vi "Facade.vi"(0 "Data In":T7 {"octave info"."engineering units" items=["custom..."=0, "V"=1, "A"=21, "C"=30, "pC"=31, "s"=32, "-"=29, "Pa"=2, "N"=20, "g"=3, "m/s^2"=4, "m/s"=5, "m"=6, "mm/s"=12, "mm"=13, "micron/s"=14, "micron"=15, "in/s^2"=7, "in/s"=8, "in"=9, "mil/s"=10, "mil"=11, "rad/s^2"=16, "rad/s"=17, "rad"=18, "deg/s^2"=26, "deg/s"=27, "deg"=28, "RPM"=22, "cycle/s^2"=23, "Hz"=24, "cycle"=25, "strain"=19]; "octave info"."dB reference" format="%.2e"; "octave info"."weighting filter" items=["Linear", "A-weighting", "B-weighting", "C-weighting", "ITU-R 468-4", "Dolby", "CCITT", "C-message", "Wb", "Wc", "Wd", "We", "Wf", "Wh", "Wj", "Wk", "Wm", "AES17 20 kHz lowpass", "AES17 40 kHz lowpass", "AES17 20 kHz highpass", "AES17 40 kHz highpass"]; "octave spectra"."band power" format="%.2f"; "octave spectra"."nominal frequencies [Hz]" format="%.2f"}, 2 "Display State In":T3={"Graph Visible Items"={"Plot Legend"=FALSE, "Scale Legend"=FALSE, "Graph Palette"=FALSE, "Cursor Legend"=FALSE, "X Scrollbar"=FALSE}, "View Table"=FALSE, "Table Visible Items"={"Vertical Scrollbar"=FALSE, "Horizontal Scrollbar"=FALSE, "Row Headers"=FALSE, "Column Headers"=FALSE, "Vertical Lines"=FALSE, "Horizontal Lines"=FALSE}, "Header Font"={"Font Name"="", "Size"=0, "Bold"=FALSE, "Italic"=FALSE, "Underline"=FALSE, "Strikeout"=FALSE, "Color"=0}, "Cell Font"={"Font Name"="", "Size"=0, "Bold"=FALSE, "Italic"=FALSE, "Underline"=FALSE, "Strikeout"=FALSE, "Color"=0}, "Description and Tip..."={"Description"="", "Tip"=""}, "Moveable Splitter Position"=0, "Measurement Cursor Configuration"={"XY"={"enable XY"=FALSE, "Position (X)"=[], "Type"=enum."Absolute", "Y reference"=0.0, "color"=0}, "band"={"enable band"=FALSE, "B1"=0.0, "B2"=0.0, "Fixed bandwidth (B2-B1)"=0.0, "B1 color"=0, "B2 color"=0}, "harmonic"={"enable harmonics"=FALSE, "X reference (1X)"=0.0, "Maximum"=0, "Subset"=enum."All", "1X color"=0, "MX color"=0}, "sideband"={"enable sideband"=FALSE, "X center (C)"=0.0, "Sidebands"=0, "X spacing (s)"=0.0, "Center color"=0, "Sideband color"=0}}, "Cursors"={"List"=[], "Tags"=[]}, "X Increment"=0.0, "X Scale"={"Label Visible"=FALSE, "Label Text"="", "Mapping Mode"=0, "Format String"=""}, "Y Scale"={"Label Visible"=FALSE, "Label Text"="", "Mapping Mode"=0, "Format String"=""}, "Colors"={"background"=16777215, "major grid"=8355711, "minor grid"=12632256, "font"=0}, "desired spectrum view"={"scaling"={"linear/dB"=enum."no change", "dB reference"=0.0, "power/magnitude"=enum."no change", "view"=enum."no change"}, "spectral density"=enum."no change"}, "Plot Color Wheel"=[3381759, 32768, 982784, 4375295, 13827953, 13457919, 16757522, 4343295, 16728758, 12095254], "Plots"=[], "registered user events"=variant, "Lock 1X to Peak"=FALSE} {"Y Scale"."Mapping Mode" items=["Linear", "Logarithmic", "dB"]; "X Scale"."Mapping Mode" items=["Linear", "Logarithmic"]}, 3 "Container State":T6) -> (6 "Data Out":T7 {"octave info"."engineering units" items=["custom..."=0, "V"=1, "A"=21, "C"=30, "pC"=31, "s"=32, "-"=29, "Pa"=2, "N"=20, "g"=3, "m/s^2"=4, "m/s"=5, "m"=6, "mm/s"=12, "mm"=13, "micron/s"=14, "micron"=15, "in/s^2"=7, "in/s"=8, "in"=9, "mil/s"=10, "mil"=11, "rad/s^2"=16, "rad/s"=17, "rad"=18, "deg/s^2"=26, "deg/s"=27, "deg"=28, "RPM"=22, "cycle/s^2"=23, "Hz"=24, "cycle"=25, "strain"=19]; "octave info"."dB reference" format="%.2e"; "octave info"."weighting filter" items=["Linear", "A-weighting", "B-weighting", "C-weighting", "ITU-R 468-4", "Dolby", "CCITT", "C-message", "Wb", "Wc", "Wd", "We", "Wf", "Wh", "Wj", "Wk", "Wm", "AES17 20 kHz lowpass", "AES17 40 kHz lowpass", "AES17 20 kHz highpass", "AES17 40 kHz highpass"]; "octave spectra"."band power" format="%.2f"; "octave spectra"."nominal frequencies [Hz]" format="%.2f"}, 7 "Display State Out":T3={"Graph Visible Items"={"Plot Legend"=FALSE, "Scale Legend"=FALSE, "Graph Palette"=FALSE, "Cursor Legend"=FALSE, "X Scrollbar"=FALSE}, "View Table"=FALSE, "Table Visible Items"={"Vertical Scrollbar"=FALSE, "Horizontal Scrollbar"=FALSE, "Row Headers"=FALSE, "Column Headers"=FALSE, "Vertical Lines"=FALSE, "Horizontal Lines"=FALSE}, "Header Font"={"Font Name"="", "Size"=0, "Bold"=FALSE, "Italic"=FALSE, "Underline"=FALSE, "Strikeout"=FALSE, "Color"=0}, "Cell Font"={"Font Name"="", "Size"=0, "Bold"=FALSE, "Italic"=FALSE, "Underline"=FALSE, "Strikeout"=FALSE, "Color"=0}, "Description and Tip..."={"Description"="", "Tip"=""}, "Moveable Splitter Position"=0, "Measurement Cursor Configuration"={"XY"={"enable XY"=FALSE, "Position (X)"=[], "Type"=enum."Absolute", "Y reference"=0.0, "color"=0}, "band"={"enable band"=FALSE, "B1"=0.0, "B2"=0.0, "Fixed bandwidth (B2-B1)"=0.0, "B1 color"=0, "B2 color"=0}, "harmonic"={"enable harmonics"=FALSE, "X reference (1X)"=0.0, "Maximum"=0, "Subset"=enum."All", "1X color"=0, "MX color"=0}, "sideband"={"enable sideband"=FALSE, "X center (C)"=0.0, "Sidebands"=0, "X spacing (s)"=0.0, "Center color"=0, "Sideband color"=0}}, "Cursors"={"List"=[], "Tags"=[]}, "X Increment"=0.0, "X Scale"={"Label Visible"=FALSE, "Label Text"="", "Mapping Mode"=0, "Format String"=""}, "Y Scale"={"Label Visible"=FALSE, "Label Text"="", "Mapping Mode"=0, "Format String"=""}, "Colors"={"background"=16777215, "major grid"=8355711, "minor grid"=12632256, "font"=0}, "desired spectrum view"={"scaling"={"linear/dB"=enum."no change", "dB reference"=0.0, "power/magnitude"=enum."no change", "view"=enum."no change"}, "spectral density"=enum."no change"}, "Plot Color Wheel"=[3381759, 32768, 982784, 4375295, 13827953, 13457919, 16757522, 4343295, 16728758, 12095254], "Plots"=[], "registered user events"=variant, "Lock 1X to Peak"=FALSE} {"Y Scale"."Mapping Mode" items=["Linear", "Logarithmic", "dB"]; "X Scale"."Mapping Mode" items=["Linear", "Logarithmic"]}, 8 "Action":T2)   [LabVIEW 2017, in "Octave with Cursors.xctl"]
doc: "This is the facade VI for the Spectral Graph with Measurement Cursors XControl.\nThe facade VI is only used within the context of the XControl."
uses:
  <vilib>/addons/_XControls/Octave with Cursors/Octave with Cursors.xctl
  <vilib>/addons/_XControls/Octave with Cursors/Controls/Data.ctl
  <vilib>/addons/_NISVFA/_Shared subVIs/Controls/svc_Octave Info.ctl
  <vilib>/addons/_NISVFA/_Shared subVIs/Controls/svc_Octave Standard.ctl
  <vilib>/addons/_NISVFA/_Shared subVIs/Controls/svc_Weighting Filter Text Ring.ctl
  <vilib>/addons/_NISVFA/_Shared subVIs/Controls/svc_Engineering Units Text Ring.ctl
  <vilib>/_xctls/Container State.ctl
  <vilib>/addons/_XControls/Octave with Cursors/Controls/State.ctl
  <vilib>/Utility/miscctls.llb/LVFontTypeDef.ctl
  <vilib>/addons/_XControls/Octave with Cursors/Controls/Measurement Cursor Configuration.ctl
  <vilib>/_xctls/Action.ctl
  <vilib>/addons/Sound and Vibration/svt_Controls/subVIs/Multiplot Octave Graph.ctl
  <vilib>/addons/_XControls/Octave with Cursors/Controls/Refnums Typedef.ctl
  <vilib>/addons/_XControls/Octave with Cursors/Controls/Spectrum XControl Events.ctl
  <vilib>/Utility/miscctls.llb/LVForegroundBackgroundColorsTypeDef.ctl
  <vilib>/addons/Sound and Vibration/svt_Octave/SVT Octave Spectrum Conversion (N Ch).vi
  <vilib>/_xctls/XControlSupport.lvlib
  <vilib>/addons/Sound and Vibration/svt_Octave/SoundVib_Octave.lvlib
panel:
  out "plot names":string[](array[string])
  in  "Focus Boolean":bool
  out "Octave graph":T1
  in  "View Table":bool=TRUE
  in  "Cursor Table":string[][](table)
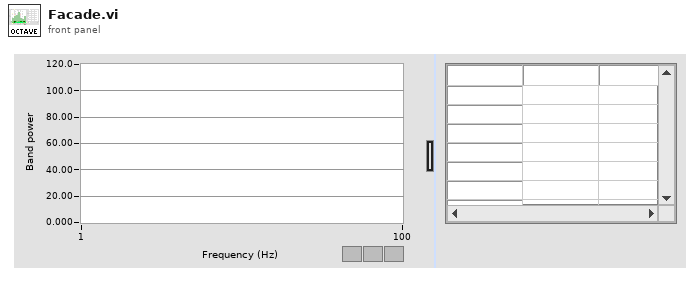
[diagram p1: front panel]
types:
  T1 = typedef "Multiplot Octave Graph.ctl" = cluster{"nominal frequencies [Hz]":dbl[], "band power [dB EU]":dbl[]}[]
  T2 = typedef "XControlSupport.lvlib/Action.ctl" = cluster{"Data Changed?":bool, "State Changed?":bool, "Action Name":string}
  T3 = typedef "Octave with Cursors.xctl/State.ctl" = cluster{"Graph Visible Items":cluster{"Plot Legend":bool, "Scale Legend":bool, "Graph Palette":bool, "Cursor Legend":bool, "X Scrollbar":bool}, "View Table":bool, "Table Visible Items":cluster{"Vertical Scrollbar":bool, "Horizontal Scrollbar":bool, "Row Headers":bool, "Column Headers":bool, "Vertical Lines":bool, "Horizontal Lines":bool}, "Header Font":T4, "Cell Font":T4, "Description and Tip...":cluster{"Description":string, "Tip":string}, "Moveable Splitter Position":i32, "Measurement Cursor Configuration":T5, "Cursors":cluster{"List":cluster{"Name":string, "Color":u32, "Style":i32, "Point Style":u8, "Name Visible":bool, "Allow Drag":bool, "Cursor Mode":u32, "Plot":i32, "Index":i32, "Position":cluster{"X":dbl, "Y":dbl}, "X Scale":u32, "Y Scale":u32, "Watch Plots":i32[], "Watch All Plots":bool, "Plot Area":i32, "Label Offset":cluster{"X":dbl, "Y":dbl}}[], "Tags":variant[]}, "X Increment":dbl, "X Scale":cluster{"Label Visible":bool, "Label Text":string, "Mapping Mode":u8, "Format String":string}, "Y Scale":cluster{"Label Visible":bool, "Label Text":string, "Mapping Mode":u8, "Format String":string}, "Colors":cluster{"background":u32, "major grid":u32, "minor grid":u32, "font":u32}, "desired spectrum view":cluster{"scaling":cluster{"linear/dB":enum16{"no change", "linear", "dB"}, "dB reference":dbl, "power/magnitude":enum16{"no change", "power", "magnitude"}, "view":enum16{"no change", "rms", "peak", "peak-peak"}}, "spectral density":enum16{"no change", "spectrum", "spectral density"}}, "Plot Color Wheel":u32[], "Plots":cluster{"Name":string, "Line Color":u32, "Line Style":u8, "Line Width":u8, "Fill/Point Color":u32, "Point Style":u8, "Fill To":i16, "Interpolation":u8, "Anti-aliased":bool}[], "registered user events":variant, "Lock 1X to Peak":bool}
  T4 = typedef "LVFontTypeDef.ctl" = cluster{"Font Name":string, "Size":u16, "Bold":bool, "Italic":bool, "Underline":bool, "Strikeout":bool, "Color":u32}
  T5 = typedef "Octave with Cursors.xctl/Measurement Cursor Configuration.ctl" = cluster{"XY":cluster{"enable XY":bool, "Position (X)":dbl[], "Type":enum16{"Absolute", "Relative"}, "Y reference":dbl, "color":u32}, "band":cluster{"enable band":bool, "B1":dbl, "B2":dbl, "Fixed bandwidth (B2-B1)":dbl, "B1 color":u32, "B2 color":u32}, "harmonic":cluster{"enable harmonics":bool, "X reference (1X)":dbl, "Maximum":i32, "Subset":enum16{"All", "Even", "Odd"}, "1X color":u32, "MX color":u32}, "sideband":cluster{"enable sideband":bool, "X center (C)":dbl, "Sidebands":i32, "X spacing (s)":dbl, "Center color":u32, "Sideband color":u32}}
  T6 = typedef "XControlSupport.lvlib/Container State.ctl" = cluster{"Indicator?":bool, "Run Mode?":bool, " Refnum":refnum<vi>}
  T7 = typedef "Octave with Cursors.xctl/Data.ctl" = cluster{"octave spectra":cluster{"nominal frequencies [Hz]":dbl[], "band power":dbl[]}[], "octave info":T8[]}
  T8 = typedef "svc_Octave Info.ctl" = cluster{"standard":T9, "bandwidth":enum16{"1 octave", "1/3 octave", "1/6 octave", "1/12 octave", "1/24 octave"}, "low band":i32, "high band":i32, "weighting filter":T10, "dB reference":dbl, "dB On":bool, "unit label":string, "channel name":string, "description":string, "engineering units":T11, "custom label":string, "spectrum type":enum16{"power", "magnitude"}, "spectral density":bool, "filters settled":bool}
  T9 = typedef "svc_Octave Standard.ctl" = enum16{"ANSI S1.11", "IEC 61260"}
  T10 = typedef "svc_Weighting Filter Text Ring.ctl" = u16
  T11 = typedef "svc_Engineering Units Text Ring.ctl" = u16
  T12 = typedef "Octave with Cursors.xctl/Refnums Typedef.ctl" = cluster{"Facade Panel Refnum":refnum<vi>, "Splitters":cluster{"Moveable":refnum<vi>, "Locked":refnum<vi>}, "Panes":cluster{"Container":refnum<vi>, "Graph":refnum<vi>, "Table":refnum<vi>, "Fixed-Width":refnum<vi>}, "Controls":cluster{"XYGraph":refnum<vi>, "Table":refnum<vi>, "View Table":refnum<vi>, "Focus Boolean":refnum<vi>, "Plot Names":refnum<vi>}}
  T13 = typedef "Octave with Cursors.xctl/Spectrum XControl Events.ctl" = string
  T14 = cluster{"linear/dB":enum16{"no change", "linear", "dB"}, "dB reference (0: no change)":dbl, "power/magnitude":enum16{"no change", "power", "magnitude"}, "spectral density":enum16{"no change", "spectrum", "spectral density"}}
  T15 = typedef "LVForegroundBackgroundColorsTypeDef.ctl" = cluster{"Foreground Color":u32, "Background Color":u32}
  T16 = cluster{"nominal frequencies [Hz]":dbl[], "band power":dbl[]}[]
  T17 = cluster{"nominal frequencies [Hz]":dbl[], "band power":dbl[]}
  T18 = typedef "eventvkey.ctl" = enum16{"ASCII", "Enter", "Return", "Shift", "Ctrl", "Alt", "Cmd", "Opt", "Caps", "NumLock", "Clear", "Break", "Up", "Down", "Left", "Right", "Insert", "Delete", "Home", "End", "PageUp", "PageDown", "Escape", "Help", "Pause", "ScrollLock", "F1", "F2", "F3", "F4", "F5", "F6", "F7", "F8", "F9", "F10", "F11", "F12", "F13", "F14", "F15", "F16", "F17", "F18", "F19", "F20", "F21", "F22", "F23", "F24", "Play", "VolumeUp", "VolumeDown", "Mute", "Two Byte Char"}
  T19 = cluster{"Shift":bool, "Ctrl":bool, "Alt":bool, "Cmd":bool, "Opt":bool}
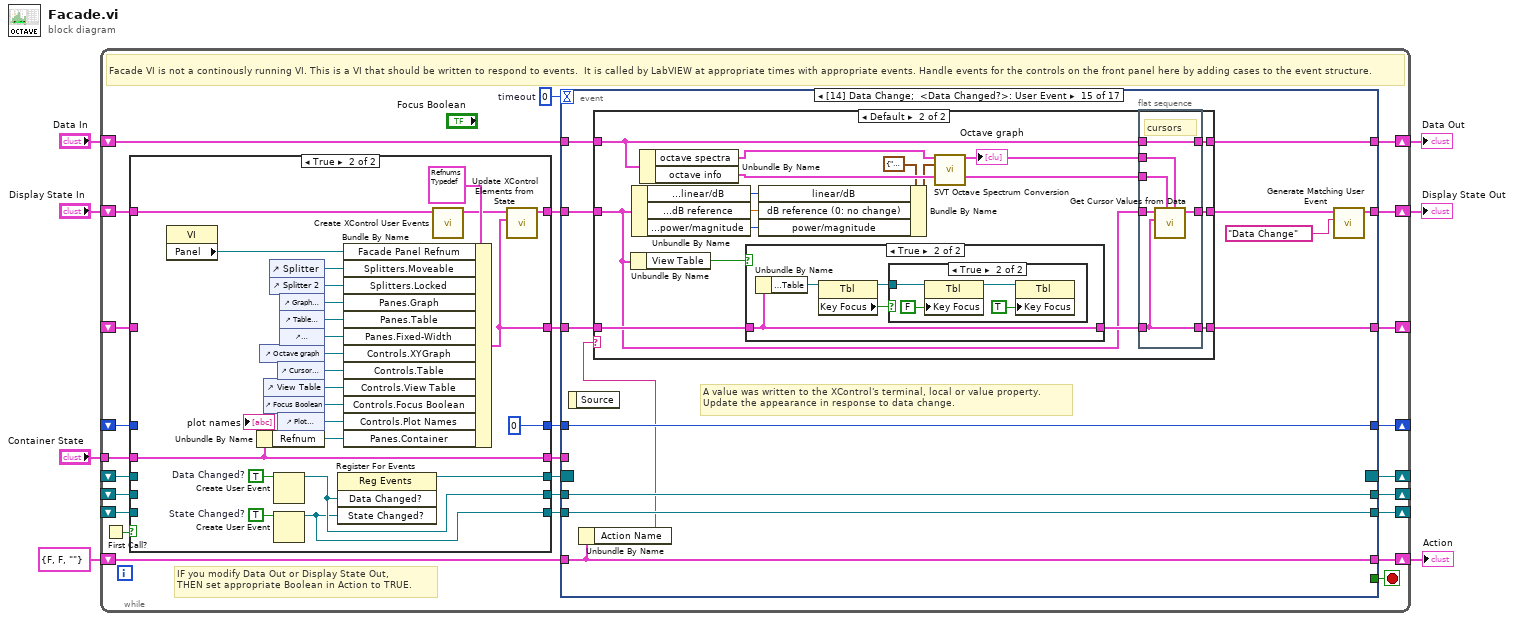
[diagram p0: block diagram]
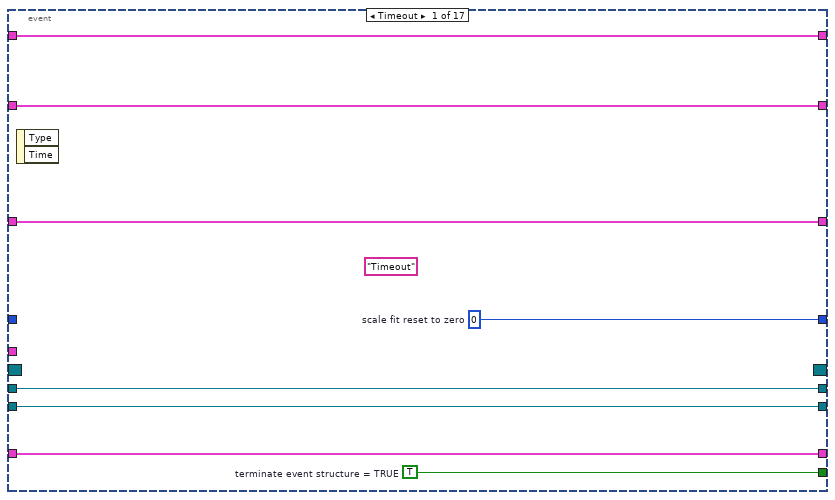
[diagram p3: hidden frame]
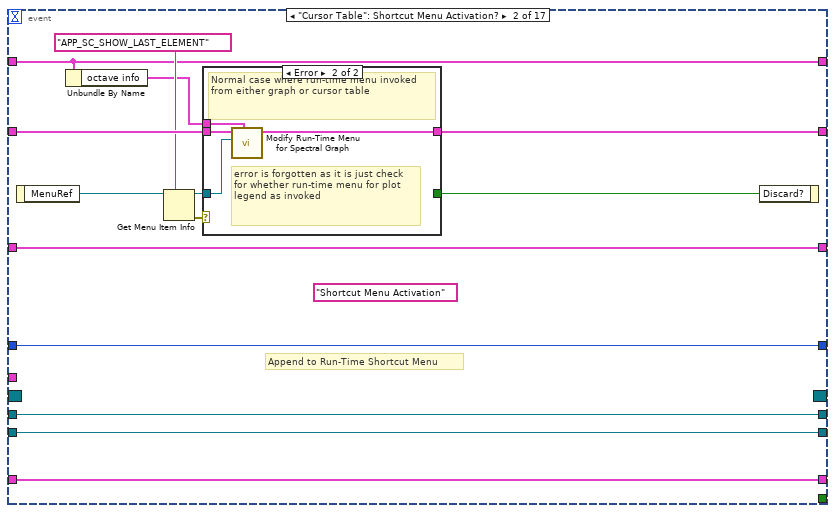
[diagram p4: hidden frame]
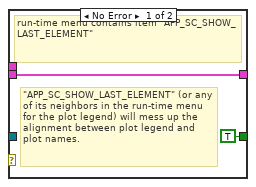
[diagram p5: hidden frame]
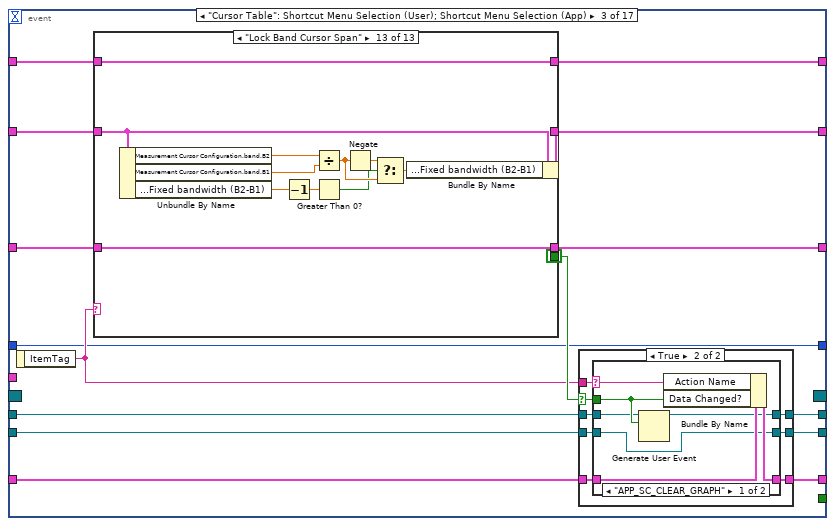
[diagram p6: hidden frame]
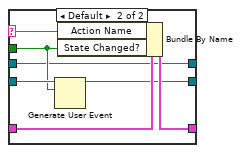
[diagram p8: hidden frame]
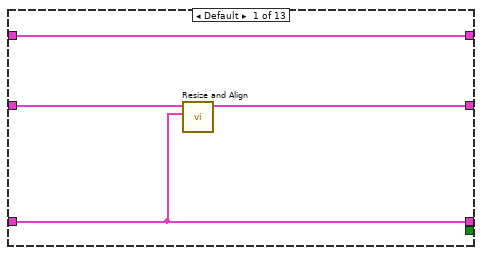
[diagram p9: hidden frame]
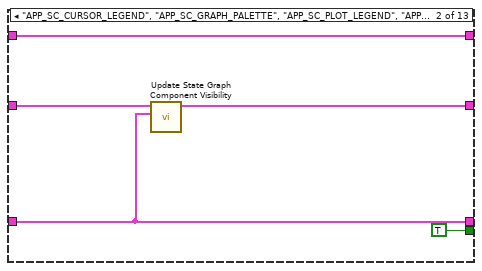
[diagram p10: hidden frame]
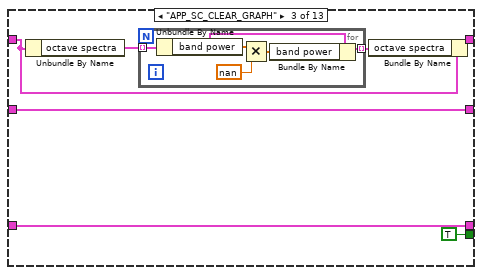
[diagram p11: hidden frame]
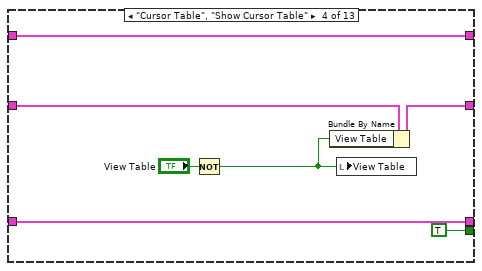
[diagram p12: hidden frame]
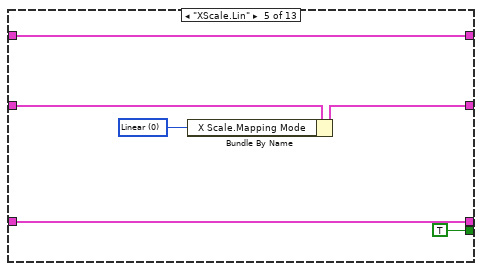
[diagram p13: hidden frame]
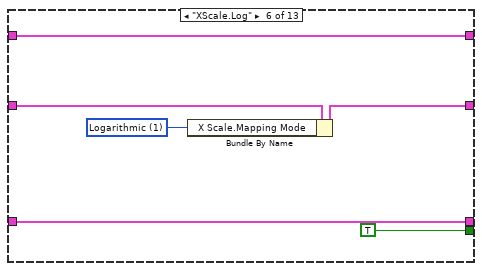
[diagram p14: hidden frame]
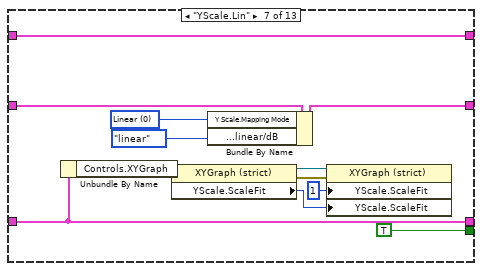
[diagram p15: hidden frame]
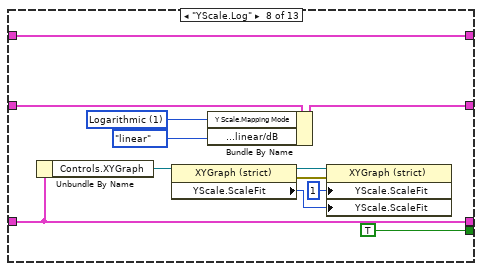
[diagram p16: hidden frame]
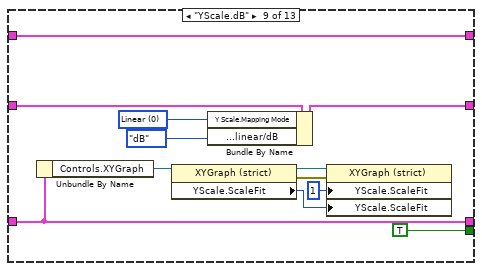
[diagram p17: hidden frame]
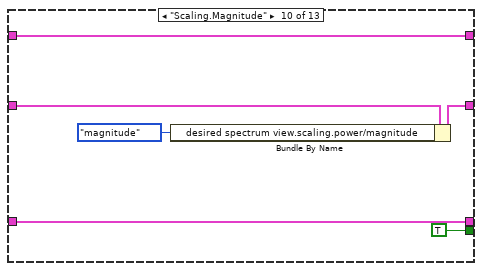
[diagram p18: hidden frame]
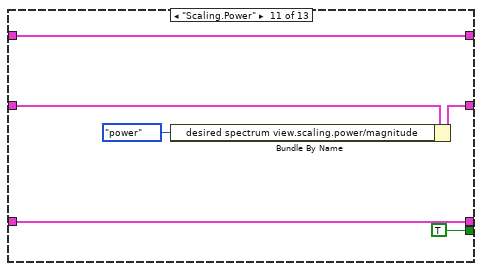
[diagram p19: hidden frame]
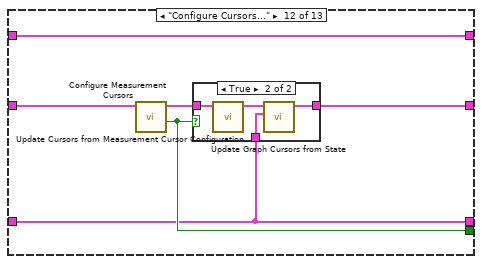
[diagram p20: hidden frame]
diagram:
  n1 = while {
    shift-right: [w28] -> w5
    shift-left: "Display State In" -> [w12]
    tunnel: "Container State" -> [w18]
    shift-right: [w32] -> w7
    shift-left: "Data In" -> [w29]
    shift-right: [w30] -> w2
    shift-left: T2 {"Data Changed?"=FALSE, "State Changed?"=FALSE, "Action Name"=""} ("Action") -> [w31]
    shift-right: [w25] -> _
    shift-left: _ -> [w23]
    shift-right: [w20] -> _
    shift-left: _ -> [w19]
    shift-right: [w24] -> _
    shift-left: _ -> [w21]
    shift-right: [w13] -> _
    shift-left: _ -> [w15]
    shift-right: [w10] -> _
    shift-left: _ -> [w9]
    stop <- w34 stop-if-true
    w33 = 0  # timeout
    # "IF you modify Data Out or Display State Out, \nTHEN set appropriate Boolean in Action to TRUE."
    # "Facade VI is not a continously running VI. This is a VI that should be written to respond to events.  It is called by LabVIEW at appropriate times with appropriate events. Handle events for the controls on the front panel here by adding cases to the event structure."
    n2 = First Call?() -> (First Call?: T/F=w22:bool)
    n3 = case shown="True" w22 {
      tunnel: [w41 w54] -> w14
      tunnel: [w40 w55] -> w27
      tunnel: [w39 w56] -> w26
      tunnel: w23 -> [w41 _]
      tunnel: w21 -> [w40 _]
      tunnel: w19 -> [w39 _]
      tunnel: w18 -> [w37 w50]
      tunnel: [w37 w50] -> w17
      tunnel: [w38 w46] -> w16
      tunnel: w15 -> [w38 _]
      tunnel: w12 -> [w35 w49]
      tunnel: [w35 w47] -> w11
      tunnel: [w36 u8 0 ("Scale Fit")] -> w8
      tunnel: w9 -> [w36 _]
      frame False {
      }
      frame True {
        w65 = TRUE  # State Changed?
        w64 = TRUE  # Data Changed?
        n4 = property class="VI"() -> ("Panel"=w45:refnum<vi>)  [unwired: 2 in, 2 out]
        n5 = Unbundle By Name(w50) -> ("Refnum"=w52:refnum<vi>)
        n6 = control-ref of="Octave graph"() -> (w43:refnum<vi>)
        n7 = control-ref of="View Table"() -> (w59:refnum<vi>)
        n8 = control-ref of="Focus Boolean"() -> (w53:refnum<vi>)
        n9 = control-ref of="Splitter"() -> (w58:refnum<vi>)
        n10 = control-ref of="Splitter 2"() -> (w57:refnum<vi>)
        n11 = Create User Event(user event datatype=w64) -> (user event=w56:refnum<user-event>)  [unwired: 1 in, 1 out]
        n12 = Create User Event(user event datatype=w65) -> (user event=w55:refnum<user-event>)  [unwired: 1 in, 1 out]
        n13 = control-ref of="Cursor Table"() -> (w60:refnum<vi>)
        n14 = control-ref of="Plot Names"() -> (w51:refnum<vi>)
        n15 = control-ref of="Graph Pane"() -> (w42:refnum<vi>)
        n16 = control-ref of="Table Pane"() -> (w62:refnum<vi>)
        n17 = control-ref of="Fixed-Width Pane"() -> (w61:refnum<vi>)
        n18 = register-events(w56, w55) -> (reference out=w54:refnum<event-registration>)  [unwired: 2 in, 1 out]
        n19 = Bundle By Name(cluster=T12 {"Facade Panel Refnum"=refnum, "Splitters"={"Moveable"=refnum, "Locked"=refnum}, "Panes"={"Container"=refnum, "Graph"=refnum, "Table"=refnum, "Fixed-Width"=refnum}, "Controls"={"XYGraph"=refnum, "Table"=refnum, "View Table"=refnum, "Focus Boolean"=refnum, "Plot Names"=refnum}} ("Refnums for Resizing and Alignment"), "Facade Panel Refnum"=w45, "Splitters.Moveable"=w58, "Splitters.Locked"=w57, "Panes.Graph"=w42, "Panes.Table"=w62, "Panes.Fixed-Width"=w61, "Controls.XYGraph"=w43, "Controls.Table"=w60, "Controls.View Table"=w59, "Controls.Focus Boolean"=w53, "Controls.Plot Names"=w51, "Panes.Container"=w52) -> (w46:T12)
        n20 = call <vilib>:"Create XControl User Events.vi"("Display State In in"=w49) -> ("Display State In out"=w44:T3)  [unwired: 9 in, 1 out]
        n21 = call <vilib>:"Update XControl Elements from State.vi"("Refnums for FP Objects"=w46, "State in"=w44) -> ("State out"=w47:T3)  [unwired: 9 in]
      }
    }
    n22 = event shown="[14] Data Change;  <Data Changed?>: User Event" {
      selector: w14 -> [_ _ _ _ _ _ _ _ _ _ _ _ _ _ _ _ _]
      dyn-events: [_ _ _ _ _ _ _ _ _ _ _ _ _ _ _ _ _] -> w25
      timeout: w33 -> [_ _ _ _ _ _ _ _ _ _ _ _ _ _ _ _ _]
      tunnel: w11 -> [w71 w83 w108 w249 w275 w286 w317 w349 w364 w377 w419 w457 w492 w508 w542 w601 w609]
      tunnel: [w71 w82 w107 w246 w274 w285 w316 w333 w363 w380 w421 w459 w491 w509 w547 w601 w609] -> w28
      tunnel: [w73 _ _ _ _ _ _ _ _ _ _ _ _ _ _ _ _] -> w34
      tunnel: w17 -> [_ _ _ _ _ _ _ _ _ _ _ _ _ _ _ w602 w610]
      tunnel: w29 -> [w70 w75 w94 w267 w284 w295 w321 w350 w368 w389 w429 w467 w497 w513 w553 w600 w608]
      tunnel: [w70 w75 w95 w267 w284 w295 w321 w350 w368 w389 w429 w467 w497 w513 w552 w600 w608] -> w32
      tunnel: [w72 w87 w105 w263 w279 w294 w320 w347 w367 w387 w427 w465 w496 w502 w544 w599 w607] -> w30
      tunnel: w31 -> [w72 w87 w106 w264 w280 w294 w320 w348 w367 w388 w428 w466 w496 w503 w544 w599 w607]
      tunnel: w16 -> [w67 w84 w100 w250 w283 w288 w318 w337 w362 w375 w417 w456 w493 w507 w546 w592 w604]
      tunnel: w26 -> [w69 w86 w101 w262 w278 w292 w313 w342 w365 w383 w423 w461 w494 w512 w545 w596 w606]
      tunnel: w27 -> [w68 w85 w104 w261 w277 w293 w312 w345 w366 w386 w426 w464 w495 w500 w543 w595 w605]
      tunnel: [w68 w85 w103 w260 w276 w293 w312 w344 w366 w385 w425 w463 w495 w499 w543 w595 w605] -> w24
      tunnel: [w69 w86 w102 w262 w278 w292 w313 w343 w365 w384 w424 w462 w494 w511 w545 w596 w606] -> w20
      tunnel: [w67 w84 w99 w250 w283 w287 w318 w337 w362 w375 w417 w456 w493 w505 w549 w592 w604] -> w13
      tunnel: [w66 w81 w96 w247 w272 w289 w310 w334 w361 w369 w410 w448 w486 w504 w551 w591 w603] -> w10
      tunnel: w8 -> [_ w81 w96 w247 w272 _ w311 w334 w361 w369 w410 w448 w486 w504 w551 w591 w603]
      event Timeout {
        w66 = u8 0  # scale fit reset to zero
        (unwired) "Timeout"
        w73 = TRUE  # terminate event structure = TRUE
        n23 = event-data() -> ()  [unwired: 1 in, 2 out]
      }
      event "Cursor Table": Shortcut Menu Activation? {
        (unwired) "Shortcut Menu Activation"
        # "Append to Run-Time Shortcut Menu"
        n24 = event-data() -> ("MenuRef"=w80:refnum<k9>)  [unwired: 1 in]
        n25 = Unbundle By Name(w75) -> ("octave info"=w74:T8[])
        n26 = Get Menu Item Info(7:"APP_SC_SHOW_LAST_ELEMENT", 11:w80) -> (0:w77:errorcluster, 3:w79:refnum<k9>)  [unwired: 1 in, 5 out]
        n27 = case shown="Error" w77 {
          tunnel: w83 -> [w89 w93]
          tunnel: [w89 w92] -> w82
          tunnel: w79 -> [_ w91]
          tunnel: [TRUE _] -> w76
          tunnel: w74 -> [_ w90]
          frame No Error {
            # "\"APP_SC_SHOW_LAST_ELEMENT\" (or any of its neighbors in the run-time menu for the plot legend) will mess up the alignment between plot legend and plot names."
            # "run-time menu contains item \"APP_SC_SHOW_LAST_ELEMENT\""
          }
          frame Error {
            # "error is forgotten as it is just check for whether run-time menu for plot legend as invoked"
            # "Normal case where run-time menu invoked from either graph or cursor table"
            n28 = call <vilib>:"Modify Run-Time Menu for Spectral Graph.vi"("octave info"=w90, "Menu in"=w91, "Display State In"=w93) -> ("Display State out"=w92:T3)  [unwired: 8 in]
          }
        }
        n29 = event-data("Discard?"=w76) -> ()  [unwired: 1 in, 1 out]
      }
      event "Cursor Table": Shortcut Menu Selection (User); Shortcut Menu Selection (App) {
        n30 = event-data() -> ("ItemTag"=w97:string)  [unwired: 1 in]
        n31 = case shown="\"Lock Band Cursor Span\"" w97 {
          tunnel: w108 -> [w137 w142 w149 w159 w166 w173 w185 w197 w209 w214 w220 w227 w237]
          tunnel: [w136 w141 w149 w158 w165 w172 w184 w196 w208 w213 w219 w225 w236] -> w107
          tunnel: [_ TRUE ("state changed") TRUE ("state changed") TRUE ("state changed") TRUE ("state changed") TRUE ("state changed") TRUE ("state changed") TRUE ("state changed") TRUE ("state changed") TRUE ("state changed") TRUE ("state changed") w224 TRUE ("state changed")] -> w98
          tunnel: w100 -> [w135 w140 w148 w161 w167 w169 w175 w187 w199 w215 w221 w223 w245]
          tunnel: [w135 w140 w148 w161 w167 w169 w175 w187 w199 w215 w221 w223 w245] -> w99
          tunnel: [w134 w138 w144 w155 w162 w168 w174 w186 w198 w210 w216 w222 w234] -> w95
          tunnel: w94 -> [w134 w138 w143 w155 w162 w168 w174 w186 w198 w210 w216 w222 w234]
          frame Default {
            n32 = call <vilib>:"Resize and Align.vi"("Refnums for Resizing and Alignment"=w135, "State in"=w137) -> ("State out"=w136:T3)  [unwired: 8 in, 1 out]
          }
          frame "APP_SC_CURSOR_LEGEND", "APP_SC_GRAPH_PALETTE", "APP_SC_PLOT_LEGEND", "APP_SC_SCALE_LEGEND", "APP_SC_X_SCALE", "APP_SC_X_SCROLLBAR", "APP_SC_Y_SCALE" {
            n33 = call <vilib>:"Update State Graph Component Visibility.vi"("Refnums for FP Objects"=w140, "State in"=w142) -> ("State out"=w141:T3)  [unwired: 9 in]
          }
          frame "APP_SC_CLEAR_GRAPH" {
            n34 = Unbundle By Name(w143) -> ("octave spectra"=w146:T16)
            n35 = for {
              tunnel: w146 -> [w152] mode=indexing
              tunnel: [w150] -> w145 mode=indexing
              n36 = Unbundle By Name(w152) -> ("band power"=w154:dbl[])
              n37 = Multiply(x=w154, y=nan) -> (x*y=w151:dbl[])
              n38 = Bundle By Name(cluster=w152, "band power"=w151) -> (w150:T17)
            }
            n39 = Bundle By Name(cluster=w143, "octave spectra"=w145) -> (w144:T7)
          }
          frame "Cursor Table", "Show Cursor Table" {
            n40 = Not(x="View Table") -> (.not. x?=w157:bool)
            n41 = Bundle By Name(cluster=w159, "View Table"=w157) -> (w158:T3)
            n42 = local write "View Table"(w157) -> ()
          }
          frame "XScale.Lin" {
            w163 = u8 0 items=["Linear", "Logarithmic"] ("Mapping Mode")
            n43 = Bundle By Name(cluster=w166, "X Scale.Mapping Mode"=w163) -> (w165:T3)
          }
          frame "XScale.Log" {
            w171 = u8 1 items=["Linear", "Logarithmic"] ("Mapping Mode")
            n44 = Bundle By Name(cluster=w173, "X Scale.Mapping Mode"=w171) -> (w172:T3)
          }
          frame "YScale.Lin" {
            w183 = u8 0 items=["Linear", "Logarithmic"] ("Mapping Mode")
            n45 = Unbundle By Name(w175) -> ("Controls.XYGraph"=w176:refnum<vi>)
            n46 = property class="XYGraph (strict)"(reference=w176) -> (reference out=w177:refnum<vi>, error out=w178:errorcluster, "YScale.ScaleFit"=w179:u8)  [unwired: 1 in]
            n47 = Bundle By Name(cluster=w185, "Y Scale.Mapping Mode"=w183, "desired spectrum view.scaling.linear/dB"=enum16{"no change", "linear", "dB"}."linear" ("spectrum view.desired scaling.linear/dB")) -> (w184:T3)
            n48 = property class="XYGraph (strict)"(reference=w177, error in=w178, "YScale.ScaleFit"=u8 1 ("Y Scale.Scale Fit"), "YScale.ScaleFit"=w179) -> ()  [unwired: 2 out]
          }
          frame "YScale.Log" {
            w194 = u8 1 items=["Linear", "Logarithmic"] ("Mapping Mode")
            n49 = Unbundle By Name(w187) -> ("Controls.XYGraph"=w188:refnum<vi>)
            n50 = property class="XYGraph (strict)"(reference=w188) -> (reference out=w189:refnum<vi>, error out=w190:errorcluster, "YScale.ScaleFit"=w191:u8)  [unwired: 1 in]
            n51 = Bundle By Name(cluster=w197, "Y Scale.Mapping Mode"=w194, "desired spectrum view.scaling.linear/dB"=enum16{"no change", "linear", "dB"}."linear" ("spectrum view.desired scaling.linear/dB")) -> (w196:T3)
            n52 = property class="XYGraph (strict)"(reference=w189, error in=w190, "YScale.ScaleFit"=u8 1 ("Y Scale.Scale Fit"), "YScale.ScaleFit"=w191) -> ()  [unwired: 2 out]
          }
          frame "YScale.dB" {
            w206 = u8 0 items=["Linear", "Logarithmic"] ("Mapping Mode")
            n53 = Unbundle By Name(w199) -> ("Controls.XYGraph"=w200:refnum<vi>)
            n54 = property class="XYGraph (strict)"(reference=w200) -> (reference out=w201:refnum<vi>, error out=w202:errorcluster, "YScale.ScaleFit"=w203:u8)  [unwired: 1 in]
            n55 = Bundle By Name(cluster=w209, "Y Scale.Mapping Mode"=w206, "desired spectrum view.scaling.linear/dB"=enum16{"no change", "linear", "dB"}."dB" ("spectrum view.desired scaling.linear/dB")) -> (w208:T3)
            n56 = property class="XYGraph (strict)"(reference=w201, error in=w202, "YScale.ScaleFit"=u8 1 ("Y Scale.Scale Fit"), "YScale.ScaleFit"=w203) -> ()  [unwired: 2 out]
          }
          frame "Scaling.Magnitude" {
            n57 = Bundle By Name(cluster=w214, "desired spectrum view.scaling.power/magnitude"=enum16{"no change", "power", "magnitude"}."magnitude") -> (w213:T3)
          }
          frame "Scaling.Power" {
            n58 = Bundle By Name(cluster=w220, "desired spectrum view.scaling.power/magnitude"=enum16{"no change", "power", "magnitude"}."power") -> (w219:T3)
          }
          frame "Configure Cursors..." {
            n59 = call <vilib>:"Configure Measurement Cursors.vi"("State in"=w227) -> ("OK"=w224:bool, "State out"=w226:T3)  [unwired: 9 in]
            n60 = case shown="True" w224 {
              tunnel: w226 -> [w228 w232]
              tunnel: [w228 w230] -> w225
              tunnel: w223 -> [_ w229]
              frame False {
              }
              frame True {
                n61 = call <vilib>:"Update Cursors from Measurement Cursor Configuration.vi"("State in"=w232) -> ("State out"=w231:T3)  [unwired: 10 in]
                n62 = call <vilib>:"Update Graph Cursors from State.vi"("Refnums for FP Objects"=w229, "State in"=w231) -> ("State out"=w230:T3)  [unwired: 9 in]
              }
            }
          }
          frame "Lock Band Cursor Span" {
            n63 = Unbundle By Name(w237) -> ("Measurement Cursor Configuration.band.B2"=w238:dbl, "Measurement Cursor Configuration.band.B1"=w239:dbl, "Measurement Cursor Configuration.band.Fixed bandwidth (B2-B1)"=w240:dbl)
            n64 = Decrement(x=w240) -> (x-1=w233:dbl)
            n65 = Divide(x=w238, y=w239) -> (x/y=w244:dbl)
            n66 = Greater Than 0?(x=w233) -> (x > 0?=w241:bool)
            n67 = Negate(x=w244) -> (-x=w242:dbl)
            n68 = Select(t=w242, s=w241, f=w244) -> (s? t:f=w243:dbl)
            n69 = Bundle By Name(cluster=w237, "Measurement Cursor Configuration.band.Fixed bandwidth (B2-B1)"=w243) -> (w236:T3)
          }
        }
        n70 = case shown="True" w98 {
          selector: w98 -> [_ w116]
          tunnel: w106 -> [w111 w119]
          tunnel: [w111 w118] -> w105
          tunnel: w97 -> [_ w114]
          tunnel: w104 -> [w110 w117]
          tunnel: [w110 w115] -> w103
          tunnel: [w109 w112] -> w102
          tunnel: w101 -> [w109 w113]
          frame False {
          }
          frame True {
            n71 = case shown="\"APP_SC_CLEAR_GRAPH\"" w114 {
              selector: w114 -> [w121 w128]
              tunnel: w119 -> [w125 w133]
              tunnel: [w124 w132] -> w118
              tunnel: w117 -> [w120 w131]
              tunnel: w116 -> [w126 w130]
              tunnel: [w120 w129] -> w115
              tunnel: w113 -> [w123 w127]
              tunnel: [w122 w127] -> w112
              frame "APP_SC_CLEAR_GRAPH" {
                n72 = Generate User Event(user event=w123, event data cluster=w126) -> (user event out=w122:refnum<user-event>)  [unwired: 2 in, 1 out]
                n73 = Bundle By Name(cluster=w125, "Action Name"=w121, "Data Changed?"=w126) -> (w124:T2)
              }
              frame Default {
                n74 = Generate User Event(user event=w131, event data cluster=w130) -> (user event out=w129:refnum<user-event>)  [unwired: 2 in, 1 out]
                n75 = Bundle By Name(cluster=w133, "Action Name"=w128, "State Changed?"=w130) -> (w132:T2)
              }
            }
          }
        }
      }
      event Pane Size {
        w248 = 10  # width - hidden splitter position
        w265 = TRUE
        n76 = event-data() -> ()  [unwired: 1 in, 1 out]
        n77 = Unbundle By Name(w250) -> ("Panes.Container"=w256:refnum<vi>, "Splitters.Moveable"=w257:refnum<vi>)
        n78 = property class="Ctl"(reference=w256) -> ("Width"=w259:u32)  [unwired: 1 in, 2 out]
        n79 = property class="Splitter"(reference=w257) -> ("Position"=w251:i32)  [unwired: 1 in, 2 out]
        n80 = Generate User Event(user event=w261, event data cluster=w265) -> (user event out=w260:refnum<user-event>)  [unwired: 2 in, 1 out]
        n81 = Bundle By Name(cluster=w264, "Action Name"="Resize", "State Changed?"=w265) -> (w263:T2)
        n82 = To Long Integer(number=w259) -> (32bit integer=w258:i32)
        n83 = Unbundle By Name(w249) -> ("View Table"=w253:bool)
        n84 = Subtract(x=w258, y=w248) -> (x-y=w255:i32)
        n85 = Not Equal?(x=w255, y=w251) -> (x != y?=w254:bool)
        n86 = And(x=w253, y=w254) -> (x .and. y?=w252:bool)
        n87 = case shown="True" w252 {
          tunnel: w249 -> [w268 w271]
          tunnel: [w268 w270] -> w246
          tunnel: w251 -> [_ w269]
          frame False {
          }
          frame True {
            n88 = Bundle By Name(cluster=w271, "Moveable Splitter Position"=w269) -> (w270:T3)
          }
        }
      }
      event "View Table": Value Change {
        w281 = TRUE
        n89 = event-data() -> ("NewVal"=w273:bool)  [unwired: 1 in]
        n90 = Bundle By Name(cluster=w275, "View Table"=w273) -> (w274:T3)
        n91 = Generate User Event(user event=w277, event data cluster=w281) -> (user event out=w276:refnum<user-event>)  [unwired: 2 in, 1 out]
        n92 = Bundle By Name(cluster=w280, "Action Name"="View Table Value Change", "State Changed?"=w281) -> (w279:T2)
      }
      event Autoscale Range Change {
        n93 = event-data() -> ("Kind"=w291:enum16{"X-Scale", "Y-Scale", "Z-Scale"}, "ScaleRef"=w290:refnum<vi>)  [unwired: 1 in]
        n94 = property class="GrphScl"(reference=w290) -> ("ScaleFit"=w289:u8)  [unwired: 1 in, 2 out]
        n95 = case shown="\"Y-Scale\"" w291 {
          tunnel: w286 -> [w297 w299]
          tunnel: [w297 w298] -> w285
          tunnel: [w296 w302] -> w287
          tunnel: w288 -> [w296 w301]
          tunnel: w289 -> [_ w300]
          frame "X-Scale", Default {
          }
          frame "Y-Scale" {
            n96 = case shown="1, 2" w300 {
              tunnel: w299 -> [w303 w309]
              tunnel: w301 -> [w304 w305]
              tunnel: [w303 w306] -> w298
              tunnel: [w304 w305] -> w302
              frame 0, Default {
                # "YScaleFit\nManual"
              }
              frame 1, 2 {
                # "YScaleFit\nAuto"
                n97 = call <vilib>:"Defer Panel Updates.vi"("Refnums for FP Objects"=w305, "State in"=w309) -> ("State out"=w308:T3)  [unwired: 8 in, 1 out]
                n98 = call <vilib>:"Adjust Cursor Y Position to Maintain Label Placement.vi"("Refnums for Resizing and Alignment"=w305, "Display State In"=w308) -> ("Display State Out"=w307:T3)  [unwired: 9 in]
                n99 = call <vilib>:"UnDefer Panel Updates.vi"("Refnums for FP Objects"=w305, "State in"=w307) -> ("State out"=w306:T3)  [unwired: 8 in, 1 out]
              }
            }
          }
        }
      }
      event Scale Range Change {
        (unwired) "Scale Range Change"
        # "this tells us if the scale range changed due to autoscale being set"
        n100 = event-data() -> ("Kind"=w315:enum16{"X-Scale", "Y-Scale", "Z-Scale"}, "ScaleRef"=w319:refnum<vi>)  [unwired: 1 in]
        n101 = case shown="0" w311 {
          selector: w311 -> [_ w323]
          tunnel: w319 -> [_ w325]
          tunnel: [_ w324] -> w314
          tunnel: [u8 0 ("Scale Fit") w323] -> w310
          frame Default {
          }
          frame 0 {
            n102 = property class="GrphScl"(reference=w325, "ScaleFit"=w323) -> (error out=w324:errorcluster)  [unwired: 1 in, 1 out]
          }
        }
        n103 = case shown="\"Y-Scale\"" w315 {
          tunnel: w318 -> [_ w327]
          tunnel: w317 -> [w326 w331]
          tunnel: [w326 w328] -> w316
          tunnel: w314 -> [_ _]
          frame Default {
          }
          frame "Y-Scale" {
            n104 = call <vilib>:"Defer Panel Updates.vi"("Refnums for FP Objects"=w327, "State in"=w331) -> ("State out"=w330:T3)  [unwired: 8 in, 1 out]
            n105 = call <vilib>:"Adjust Cursor Y Position to Maintain Label Placement.vi"("Refnums for Resizing and Alignment"=w327, "Display State In"=w330) -> ("Display State Out"=w329:T3)  [unwired: 9 in]
            n106 = call <vilib>:"UnDefer Panel Updates.vi"("Refnums for FP Objects"=w327, "State in"=w329) -> ("State out"=w328:T3)  [unwired: 8 in, 1 out]
          }
        }
      }
      event Cursor Move; Cursor Grab {
        n107 = event-data() -> ("CursRef"=w340:refnum<vi>, "CursLoc"=w341:cluster{"X":dbl, "Y":dbl})  [unwired: 1 in]
        n108 = property class="Curs"(reference=w340) -> ("Cursor Name"=w339:string)  [unwired: 1 in, 2 out]
        n109 = Unbundle By Name(w341) -> ("X"=w338:dbl)
        n110 = call <vilib>:"Move Set on Cursor Move.vi"("Cursor.Position.X"=w338, "Cursor Name"=w339, "Refnums for Resizing and Alignment"=w337, "Display State In"=w349) -> ("state changed"=w332:bool, "Display State Out"=w333:T3)  [unwired: 5 in, 1 out]
        n111 = Unbundle By Name(w337) -> ("Controls.Focus Boolean"=w336:refnum<vi>)
        n112 = property class="Bool (strict)"(reference=w336, "Key Focus"=TRUE) -> ()  [unwired: 1 in, 2 out]
        n113 = case shown="True" w332 {
          selector: w332 -> [_ w356]
          tunnel: w348 -> [w353 w360]
          tunnel: [w353 w359] -> w347
          tunnel: "Cursor Move" -> [_ w358]
          tunnel: w345 -> [w352 w357]
          tunnel: [w352 w355] -> w344
          tunnel: [w351 w354] -> w343
          tunnel: w342 -> [w351 w354]
          frame False {
          }
          frame True {
            n114 = Generate User Event(user event=w357, event data cluster=w356) -> (user event out=w355:refnum<user-event>)  [unwired: 2 in, 1 out]
            n115 = Bundle By Name(cluster=w360, "Action Name"=w358, "State Changed?"=w356) -> (w359:T2)
          }
        }
      }
      event Plot Attribute Change {
        n116 = event-data() -> ()  [unwired: 1 in, 2 out]
        n117 = call <vilib>:"Update State Plot Properties.vi"("Refnums for FP Objects"=w362, "State in"=w364) -> ("State out"=w363:T3)  [unwired: 9 in]
      }
      event "Cursor Table": Value Change {
        n118 = event-data() -> ("NewVal"=w382:string[][], "OldVal"=w370:string[][], "CtlRef"=w371:refnum<vi>)  [unwired: 1 in]
        n119 = call <vilib>:"Verify New Value is Valid X.vi"("OldVal"=w370, "NewVal"=w382, "Refnums for Resizing and Alignment"=w375, "State in"=w377) -> ("X position"=w372:dbl, "cursor name"=w373:string, "Refnums for Resizing and Alignment out"=w374:T12, "State out"=w376:T3, "valid X change"=w379:bool)  [unwired: 3 in]
        n120 = case shown="True" w379 {
          selector: w379 -> [w390 _]
          tunnel: w374 -> [_ w397]
          tunnel: w376 -> [w391 w396]
          tunnel: [w391 w392] -> w380
          tunnel: [w390 w393] -> w378
          tunnel: w373 -> [_ w395]
          tunnel: w372 -> [_ w394]
          frame False {
          }
          frame True {
            n121 = call <vilib>:"Move Set on Cursor Move.vi"("Cursor.Position.X"=w394, "Cursor Name"=w395, "Refnums for Resizing and Alignment"=w397, "Display State In"=w396) -> ("state changed"=w393:bool, "Display State Out"=w392:T3)  [unwired: 5 in, 1 out]
          }
        }
        n122 = case shown="False" w378 {
          selector: w378 -> [_ w403]
          tunnel: w388 -> [w402 w409]
          tunnel: [w402 w408] -> w387
          tunnel: "Cursor Table Value Change" -> [_ w407]
          tunnel: w386 -> [w401 w406]
          tunnel: [w401 w405] -> w385
          tunnel: [w400 w404] -> w384
          tunnel: w383 -> [w400 w404]
          tunnel: w371 -> [w399 _]
          tunnel: w370 -> [w398 _]
          frame False {
            n123 = property on="Property Node" class="Tbl (strict)"(reference=w399, "Value"=w398) -> ()  [unwired: 1 in, 2 out]
          }
          frame True {
            n124 = Bundle By Name(cluster=w409, "State Changed?"=w403, "Action Name"=w407) -> (w408:T2)
            n125 = Generate User Event(user event=w406, event data cluster=w403) -> (user event out=w405:refnum<user-event>)  [unwired: 2 in, 1 out]
          }
        }
      }
      event "Cursor Table", "Focus Boolean": Key Down? {
        n126 = event-data() -> ("VKey"=w420:T18, "PlatMods"=w413:T19)  [unwired: 1 in]
        n127 = call <vilib>:"Update Control Based on Key Down.vi"("PlatMods"=w413, "VKey"=w420, "Refnums for Resizing and Alignment in"=w417, "display state in"=w419) -> ("Position.X"=w414:dbl, "selected cursor"=w415:string, "Refnums for Resizing and Alignment out"=w416:T12, "display state out"=w418:T3, "discard?"=w411:bool)  [unwired: 3 in]
        n128 = case shown="True" w411 {
          selector: w411 -> [w430 _]
          tunnel: w416 -> [_ w437]
          tunnel: w418 -> [w431 w436]
          tunnel: [w431 w432] -> w421
          tunnel: [w430 w433] -> w412
          tunnel: w415 -> [_ w435]
          tunnel: w414 -> [_ w434]
          frame False {
          }
          frame True {
            n129 = call <vilib>:"Move Set on Cursor Move.vi"("Cursor.Position.X"=w434, "Cursor Name"=w435, "Refnums for Resizing and Alignment"=w437, "Display State In"=w436) -> ("state changed"=w433:bool, "Display State Out"=w432:T3)  [unwired: 5 in, 1 out]
          }
        }
        n130 = case shown="True" w412 {
          selector: w412 -> [_ w441]
          tunnel: w428 -> [w440 w447]
          tunnel: [w440 w446] -> w427
          tunnel: "Cursor Move" -> [_ w445]
          tunnel: w426 -> [w439 w444]
          tunnel: [w439 w443] -> w425
          tunnel: [w438 w442] -> w424
          tunnel: w423 -> [w438 w442]
          frame False {
          }
          frame True {
            n131 = Bundle By Name(cluster=w447, "State Changed?"=w441, "Action Name"=w445) -> (w446:T2)
            n132 = Generate User Event(user event=w444, event data cluster=w441) -> (user event out=w443:refnum<user-event>)  [unwired: 2 in, 1 out]
          }
        }
        n133 = event-data("Discard?"=w411) -> ()  [unwired: 1 in, 1 out]
      }
      event "Cursor Table", "Focus Boolean": event type 3.0.x8000000b {
        n134 = event-data() -> ("VKey"=w453:T18, "PlatMods"=w454:T19)  [unwired: 1 in]
        n135 = call <vilib>:"Update Control Based on Key Down.vi"("PlatMods"=w454, "VKey"=w453, "Refnums for Resizing and Alignment in"=w456, "display state in"=w457) -> ("Position.X"=w449:dbl, "selected cursor"=w450:string, "Refnums for Resizing and Alignment out"=w451:T12, "display state out"=w452:T3, "discard?"=w455:bool)  [unwired: 3 in]
        n136 = case shown="True" w455 {
          selector: w455 -> [w468 _]
          tunnel: w451 -> [_ w475]
          tunnel: w452 -> [w469 w474]
          tunnel: [w469 w470] -> w459
          tunnel: [w468 w471] -> w458
          tunnel: w450 -> [_ w473]
          tunnel: w449 -> [_ w472]
          frame False {
          }
          frame True {
            n137 = call <vilib>:"Move Set on Cursor Move.vi"("Cursor.Position.X"=w472, "Cursor Name"=w473, "Refnums for Resizing and Alignment"=w475, "Display State In"=w474) -> ("state changed"=w471:bool, "Display State Out"=w470:T3)  [unwired: 5 in, 1 out]
          }
        }
        n138 = case shown="True" w458 {
          selector: w458 -> [_ w479]
          tunnel: w466 -> [w478 w485]
          tunnel: [w478 w484] -> w465
          tunnel: "Cursor Move" -> [_ w483]
          tunnel: w464 -> [w477 w482]
          tunnel: [w477 w481] -> w463
          tunnel: [w476 w480] -> w462
          tunnel: w461 -> [w476 w480]
          frame False {
          }
          frame True {
            n139 = Bundle By Name(cluster=w485, "State Changed?"=w479, "Action Name"=w483) -> (w484:T2)
            n140 = Generate User Event(user event=w482, event data cluster=w479) -> (user event out=w481:refnum<user-event>)  [unwired: 2 in, 1 out]
          }
        }
        n141 = event-data("Discard?"=w455) -> ()  [unwired: 1 in, 1 out]
      }
      event "Cursor Table": Mouse Down {
        (unwired) "Cursor Table Mouse Down" ("ItemTag")
        n142 = event-data() -> ("Coords.Horizontal"=w490:i32, "Coords.Vertical"=w489:i32)  [unwired: 1 in]
        n143 = Bundle By Name(cluster=cluster{"horizontal":i32, "vertical":i32} {"horizontal"=0, "vertical"=0} ("Point"), "horizontal"=w490, "vertical"=w489) -> (w487:cluster{"horizontal":i32, "vertical":i32})
        n144 = call <vilib>:"Set Active Cursor from Table.vi"("Point"=w487, "Refnums for Resizing and Alignment"=w493, "Display State In"=w492) -> ("Display State Out"=w491:T3)  [unwired: 8 in]
      }
      event Display State Change; User Event {
        w501 = T13 "Display State Change"
        # "Display State changed as a result of dropping a new instance of this XControl, copying, undoing an operation or executing a custom property or method on this XControl. Update the appearance accordingly."
        n145 = event-data() -> ()  [unwired: 1 in, 3 out]
        n146 = Unbundle By Name(w503) -> ("Action Name"=w506:string)
        n147 = case shown="Default" w506 {
          selector: w506 -> [_ _ w536]
          tunnel: [w526 w528 w529] -> w510
          tunnel: w508 -> [w526 w528 w532]
          tunnel: w507 -> [w525 w527 w533]
          tunnel: [w525 w527 w533] -> w505
          tunnel: [TRUE ("Data Changed?") _ w535] -> w498
          frame "Cursor Move", "Lock 1X to Peak", "Snap 1X to Peak" {
          }
          frame "1X Cursor Track" {
          }
          frame Default {
            n148 = call <vilib>:"Defer Panel Updates.vi"("Refnums for FP Objects"=w533, "State in"=w532) -> ("State out"=w530:T3)  [unwired: 8 in, 1 out]
            n149 = call <vilib>:"Update Graph Cursors from State.vi"("Refnums for FP Objects"=w533, "State in"=w530) -> ("State out"=w537:T3)  [unwired: 9 in]
            n150 = call <vilib>:"Set Graph Scale Properties.vi"("Refnums in"=w533, "Display State In"=w537) -> ("Display State out"=w539:T3)  [unwired: 9 in]
            n151 = call <vilib>:"Resize and Align.vi"("Refnums for Resizing and Alignment"=w533, "State in"=w539) -> ("State out"=w538:T3)  [unwired: 8 in, 1 out]
            n152 = call <vilib>:"Adjust Cursor Y Position to Maintain Label Placement.vi"("Refnums for Resizing and Alignment"=w533, "Display State In"=w538) -> ("Display State Out"=w540:T3)  [unwired: 9 in]
            n153 = call <vilib>:"Set Colors.vi"("Refnums"=w533, "Display State In"=w540) -> ("Display State Out"=w531:T3)  [unwired: 9 in]
            n154 = Not Equal?(x="Resize", y=w536) -> (x != y?=w535:bool)
            n155 = call <vilib>:"UnDefer Panel Updates.vi"("Refnums for FP Objects"=w533, "State in"=w531) -> ("State out"=w529:T3)  [unwired: 8 in, 1 out]
          }
        }
        n156 = case shown="True" w498 {
          selector: w498 -> [_ w517]
          tunnel: w512 -> [w515 w523]
          tunnel: [w515 w522] -> w511
          tunnel: w503 -> [w514 w521]
          tunnel: [w514 w520] -> w502
          tunnel: w501 -> [_ w519]
          tunnel: [w516 w518] -> w499
          tunnel: w500 -> [w516 w518]
          frame False {
          }
          frame True {
            n157 = Bundle By Name(cluster=w521, "Action Name"=w519, "Data Changed?"=w517) -> (w520:T2)
            n158 = Generate User Event(user event=w523, event data cluster=w517) -> (user event out=w522:refnum<user-event>)  [unwired: 2 in, 1 out]
          }
        }
        n159 = call <vilib>:"Generate Matching User Event.vi"("event"=w501, "Display State in"=w510) -> ("Display State out"=w509:T3)  [unwired: 8 in, 1 out]
      }
      event Data Change; User Event {
        # "A value was written to the XControl's terminal, local or value property.\nUpdate the appearance in response to data change."
        n160 = event-data() -> ()  [unwired: 1 in, 1 out]
        n161 = Unbundle By Name(w544) -> ("Action Name"=w541:string)
        n162 = case shown="Default" w541 {
          tunnel: w553 -> [w554 w568]
          tunnel: [w554 w575] -> w552
          tunnel: [w558 w574] -> w549
          tunnel: [w557 w573] -> w548
          tunnel: w546 -> [w558 w572]
          tunnel: w542 -> [w557 w560]
          frame "APP_SC_CLEAR_GRAPH" {
            n163 = Unbundle By Name(w554) -> ("octave spectra"=w555:T16)
            n164 = local write "Cursor Table"(string[][] [[" "]] ("Cursor Table")) -> ()
            n165 = local write "Octave graph"(w555) -> ()
          }
          frame Default {
            n166 = Unbundle By Name(w560) -> ("View Table"=w570:bool)
            n167 = Unbundle By Name(w560) -> ("desired spectrum view.scaling.linear/dB"=w563:enum16{"no change", "linear", "dB"}, "desired spectrum view.scaling.dB reference"=w562:dbl, "desired spectrum view.scaling.power/magnitude"=w561:enum16{"no change", "power", "magnitude"})
            n168 = Unbundle By Name(w568) -> ("octave spectra"=w559:T16, "octave info"=w569:T8[])
            n169 = case shown="True" w570 {
              tunnel: w572 -> [w576 w577]
              tunnel: [w576 w577] -> w571
              frame False {
              }
              frame True {
                n170 = Unbundle By Name(w577) -> ("Controls.Table"=w580:refnum<vi>)
                n171 = property class="Tbl"(reference=w580) -> (reference out=w578:refnum<vi>, "Key Focus"=w579:bool)  [unwired: 1 in, 1 out]
                n172 = case shown="True" w579 {
                  tunnel: w578 -> [_ w583]
                  frame False {
                  }
                  frame True {
                    n173 = property class="Tbl"(reference=w583, "Key Focus"=FALSE) -> (reference out=w582:refnum<vi>)  [unwired: 1 in, 1 out]
                    n174 = property class="Tbl"(reference=w582, "Key Focus"=TRUE) -> ()  [unwired: 1 in, 2 out]
                  }
                }
              }
            }
            n175 = Bundle By Name(cluster=T14 {"linear/dB"=enum."no change", "dB reference (0: no change)"=0.0, "power/magnitude"=enum."no change", "spectral density"=enum."no change"} ("desired scaling"), "linear/dB"=w563, "dB reference (0: no change)"=w562, "power/magnitude"=w561) -> (w564:T14)
            n176 = call-poly <vilib>:"SVT Octave Spectrum Conversion.vi"("octave spectra"=w559, "desired scaling"=w564, "octave info in"=w569) -> ("converted octave spectra"=w567:T16, "octave info out"=w566:T8[])  [unwired: 9 in, 2 out]
            "Octave graph" <- w567
            n177 = flat-sequence {
              tunnel: w560 -> [w590]
              tunnel: w571 -> [w586]
              tunnel: w566 -> [w589]
              tunnel: w567 -> [w588]
              tunnel: w568 -> [w587]
              tunnel: [w587] -> w575
              tunnel: [w586] -> w574
              tunnel: [w585] -> w573
              frame #0 {
                # "cursors"
                n178 = call <vilib>:"Get Cursor Values from Data.vi"("octave spectra"=w588, "octave info"=w589, "Refnums for FP Objects"=w586, "Display State In"=w590) -> ("Display State Out"=w585:T3)  [unwired: 4 in, 3 out]
              }
            }
          }
        }
        n179 = call <vilib>:"Generate Matching User Event.vi"("event"=T13 "Data Change", "Display State in"=w548) -> ("Display State out"=w547:T3)  [unwired: 8 in, 1 out]
      }
      event Direction Change {
        (unwired) "Direction Change"
        # "The direction of the XControl changed from a control to an indicator or vice versa. Update the appearance accordingly."
        n180 = event-data() -> ()  [unwired: 1 in, 4 out]
        n181 = Unbundle By Name(w592) -> ("Splitters.Locked"=w598:refnum<vi>)
        n182 = Unbundle By Name(w602) -> ("Refnum"=w594:refnum<vi>)
        n183 = property class="Splitter"(reference=w598, "Colors"=T15 {"Foreground Color"=16777216, "Background Color"=16777216}) -> ()  [unwired: 1 in, 2 out]
        n184 = property class="Ctl"(reference=w594, "SyncDisp"=TRUE ("Synchronous Display")) -> ()  [unwired: 1 in, 2 out]
      }
      event Exec State Change {
        (unwired) "Exec State Change"
        # "The VI owning the XControl changed from Edit Mode  to Run Mode or vice versa.\nUpdate the appearance accordingly."
        # "Handle Edit Mode & Run Mode\ncase differently"
        n185 = event-data() -> ()  [unwired: 1 in, 4 out]
        n186 = Unbundle By Name(w610) -> ()  [unwired: 1 out]
      }
    }
  }
  "Display State Out" <- w5
  "Data Out" <- w7
  "Action" <- w2
